vi "Json Token to Cluster Data.vi"(0 "Token Array":T1[](array[typedef]), 1 "Variable Names":string[](array[string]), 5 "Index":i32, 7 "Parent Ref In":refnum<vi>[](array[refnum]), 9 "Inception Tracking In":cluster{"In Array?":bool, "Cluster Level":i32}={"In Array?"=TRUE, "Cluster Level"=0}, 11 "Error In":errorcluster) -> (4 "index out":i32, 6 "Parent Ref Out":refnum<vi>[](array[refnum]), 10 "Inception Tracking Out":cluster{"In Array?":bool, "Cluster Level":i32}={"In Array?"=TRUE, "Cluster Level"=0}, 14 "End?":bool, 15 "Error Out":errorcluster)   [LabVIEW 2019, in "SLL JSON to Cluster.lvlib"]
doc: "This VI converts input JSON tokens to its equivalent cluster data"
uses:
  SLL JSON to Cluster.lvlib
  _Controls/Tokens.ctl
  <vilib>/numeric/LVNumericRepresentation.ctl
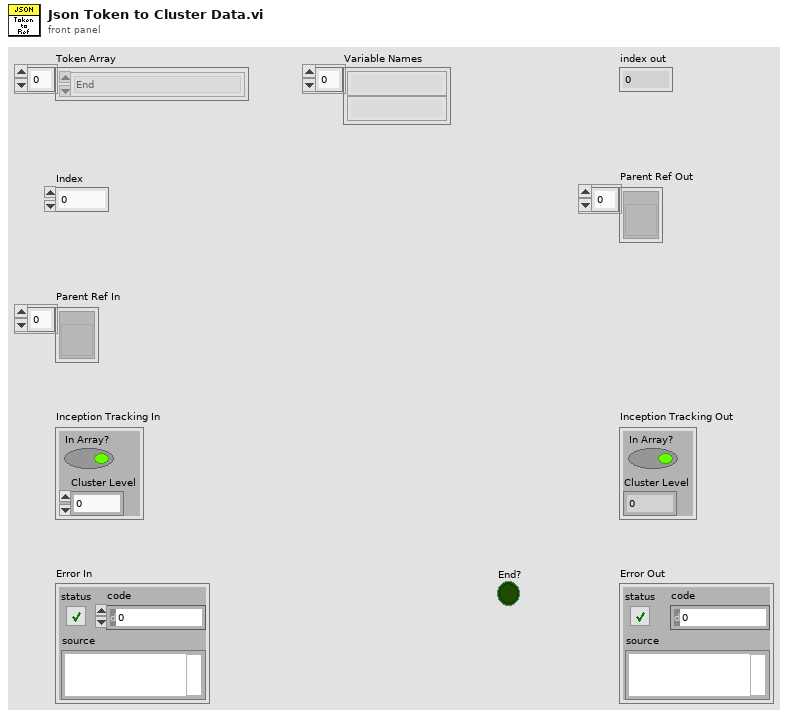
[diagram p1: front panel]
types:
  T1 = typedef "SLL JSON to Cluster.lvlib/Tokens.ctl" = enum16{"End", "Boolean", "Named Cluster", "Unnamed Cluster", "Array", "String", "Decimal", "FloatingPoint", "End Array", "End Cluster"}
  T2 = typedef "LVNumericRepresentation.ctl" = enum32{"Extended Precision", "Double Precision", "Single Precision", "Long", "Word", "Byte", "Unsigned Long", "Unsigned Word", "Unsigned Byte", "Complex Extended", "Complex Double", "Complex Single", "Quad", "Unsigned Quad", "Fixed-Point"}
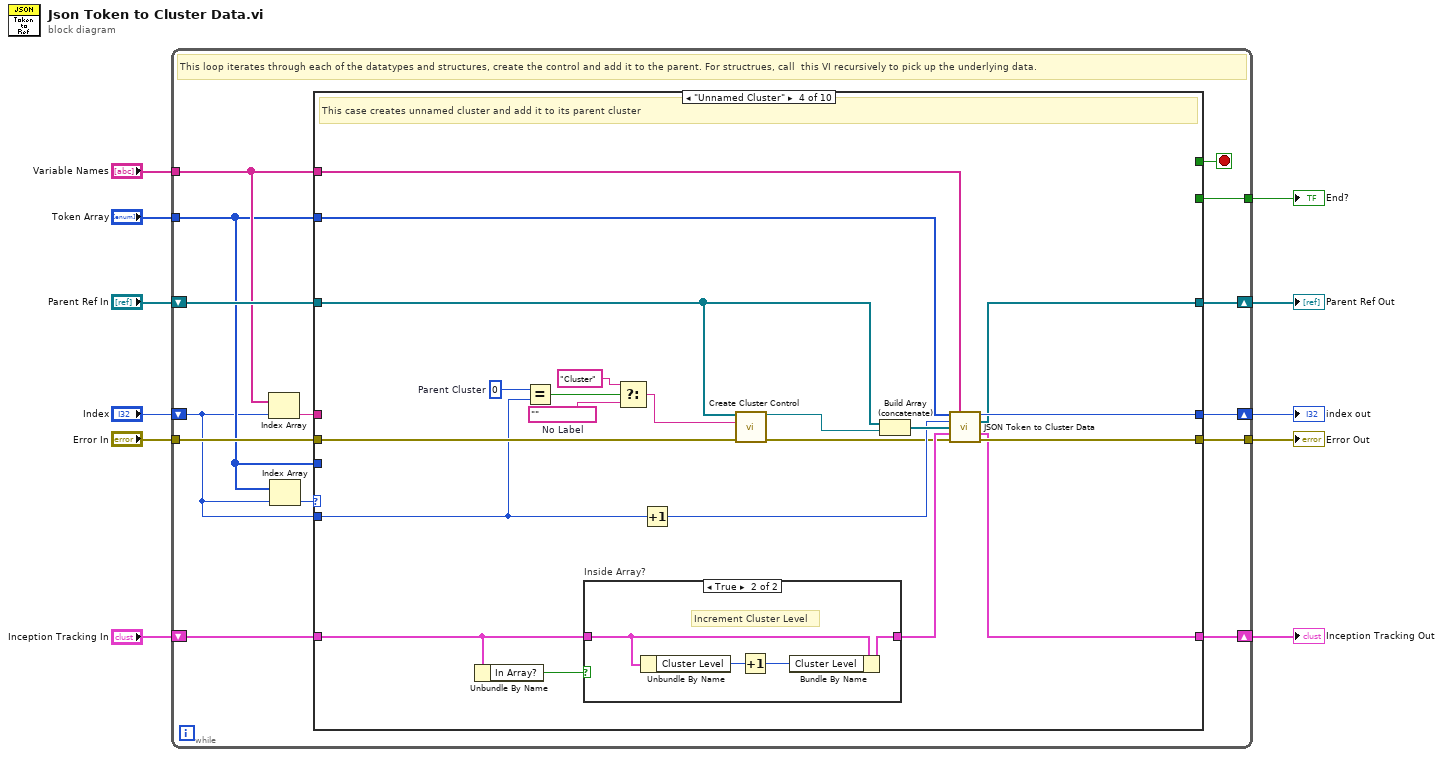
[diagram p0: block diagram]
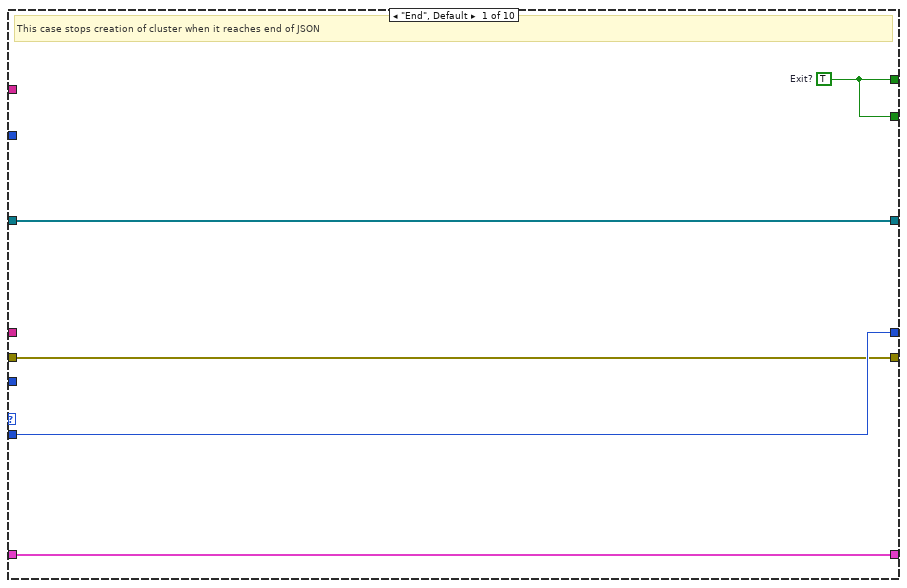
[diagram p2: hidden frame]
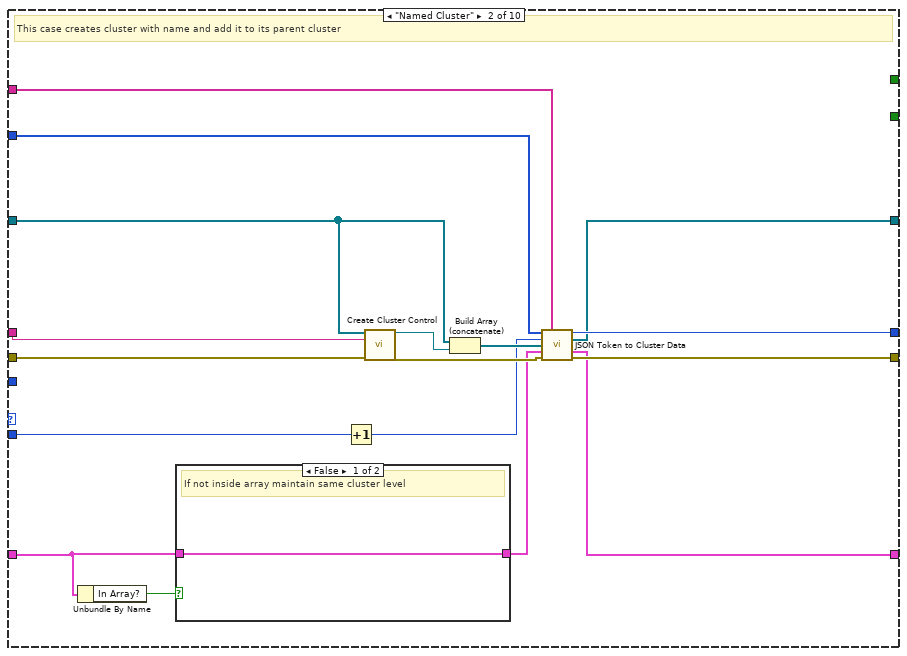
[diagram p3: hidden frame]
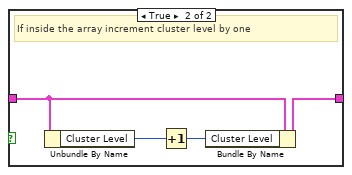
[diagram p4: hidden frame]
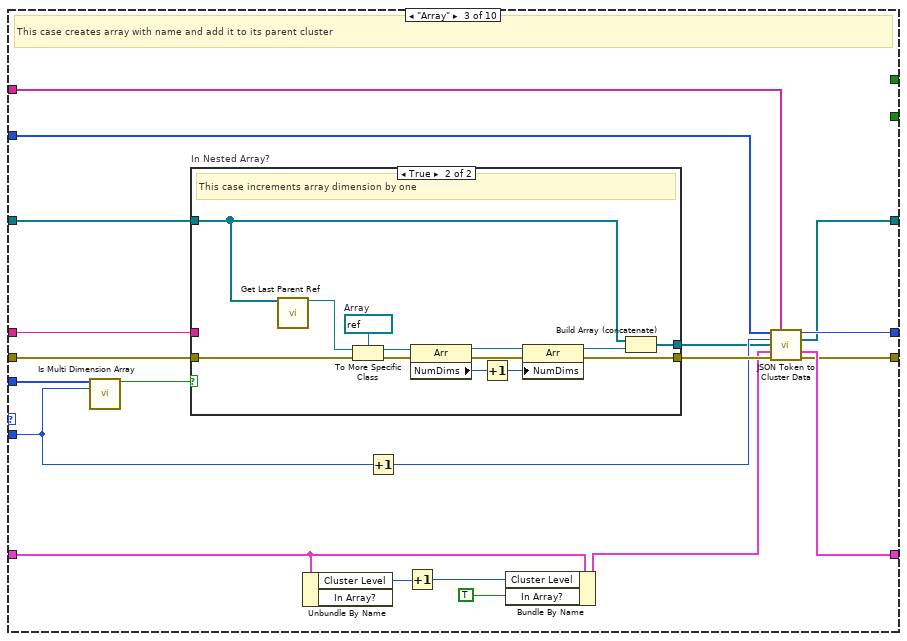
[diagram p5: hidden frame]
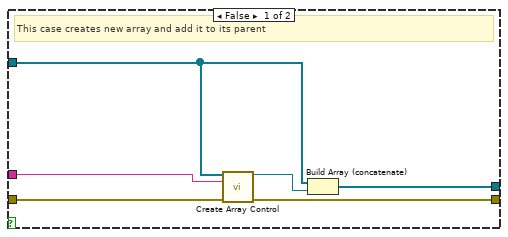
[diagram p6: hidden frame]
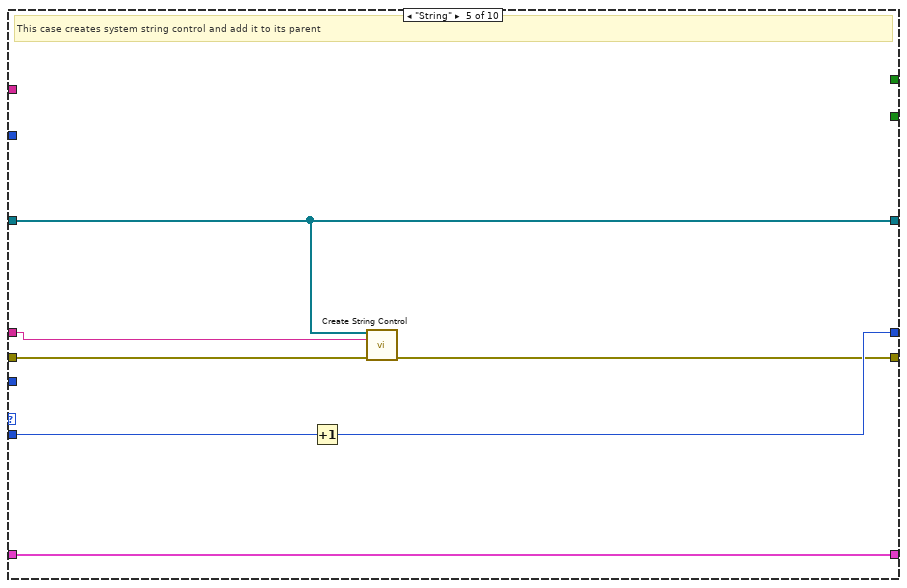
[diagram p8: hidden frame]
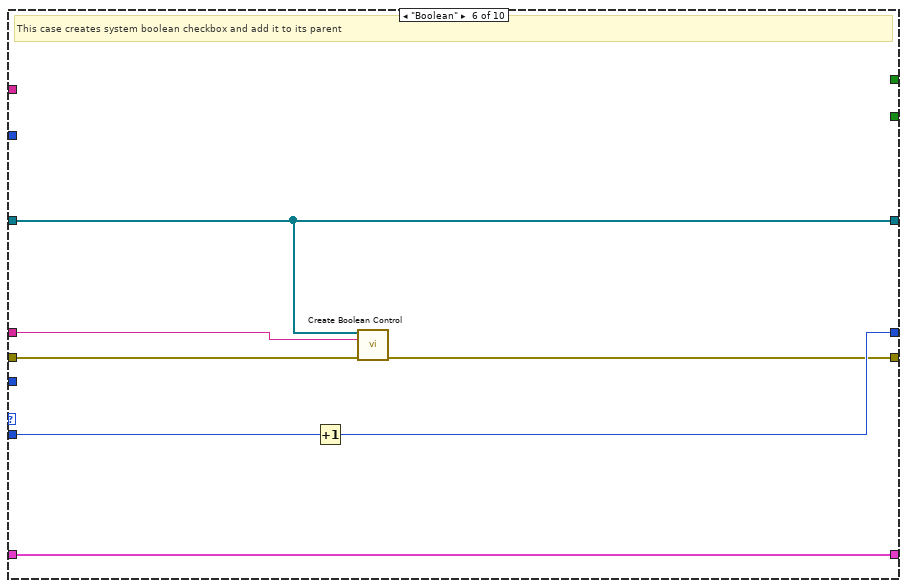
[diagram p9: hidden frame]
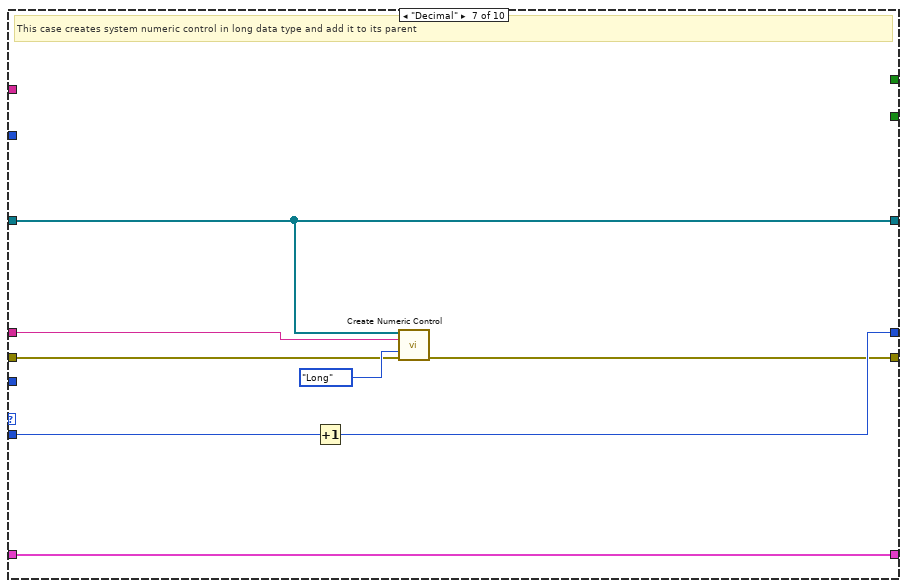
[diagram p10: hidden frame]
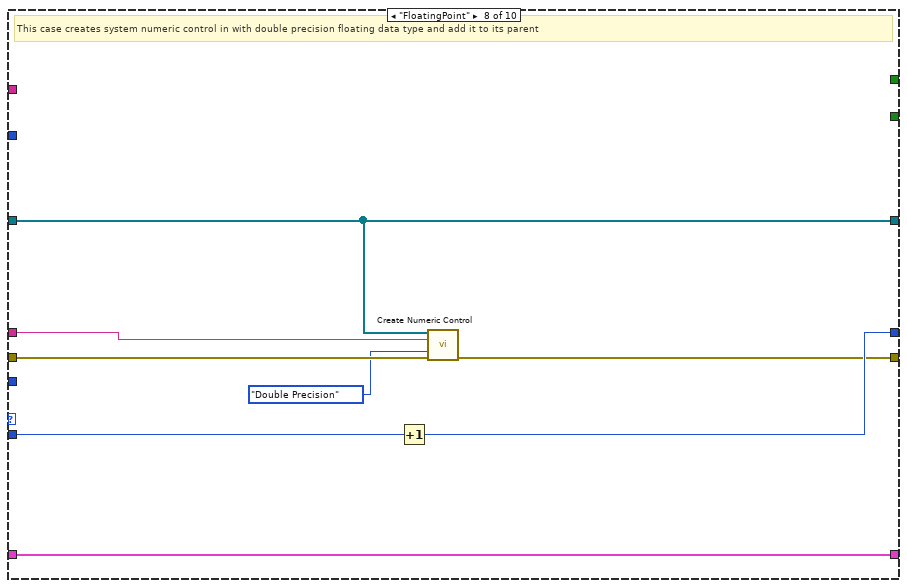
[diagram p11: hidden frame]
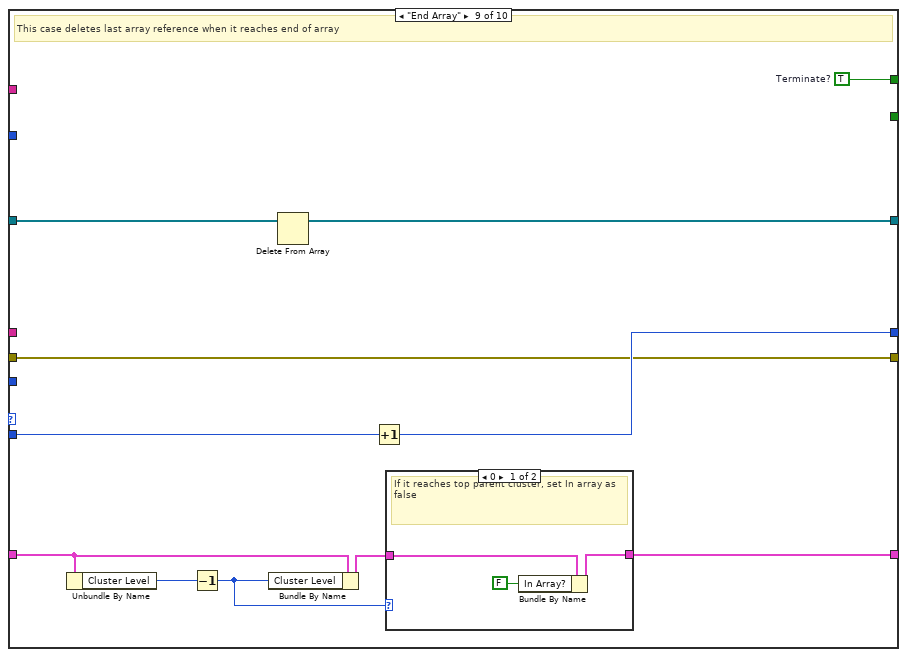
[diagram p12: hidden frame]
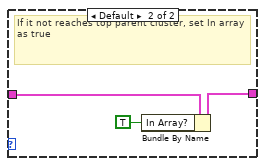
[diagram p13: hidden frame]
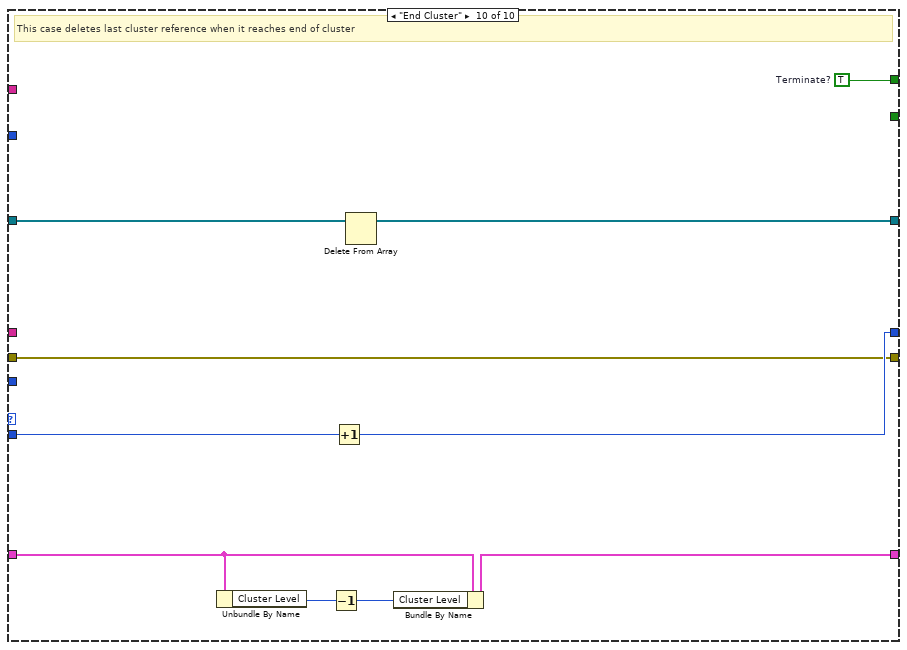
[diagram p14: hidden frame]
diagram:
  n1 = while {
    tunnel: "Token Array" -> [w13]
    shift-right: [w21] -> w9
    shift-left: "Index" -> [w12]
    shift-right: [w22] -> w4
    shift-left: "Parent Ref In" -> [w24]
    tunnel: "Variable Names" -> [w18]
    tunnel: [w19] -> w7
    shift-right: [w16] -> w5
    shift-left: "Inception Tracking In" -> [w17]
    tunnel: "Error In" -> [w15]
    tunnel: [w14] -> w1
    stop <- w20 stop-if-true
    # "This loop iterates through each of the datatypes and structures, create the control and add it to the parent. For structrues, call  this VI recursively to pick up the underlying data."
    n2 = Index Array(array=w18, index=w12) -> (element=w23:string)
    n3 = Index Array(array=w13, index=w12) -> (element=w25:T1)
    n4 = case shown="\"Unnamed Cluster\"" w25 {
      tunnel: w24 -> [w29 w43 w71 w100 w118 w125 w132 w141 w150 w167]
      tunnel: w23 -> [_ w46 w72 _ w124 w131 w137 w140 _ _]
      tunnel: [w29 w33 w61 w102 w118 w125 w132 w141 w149 w166] -> w22
      tunnel: w12 -> [w28 w47 w54 w97 w123 w130 w139 w147 w157 w173]
      tunnel: [w28 w34 w64 w104 w122 w129 w138 w146 w156 w172] -> w21
      tunnel: [w30 _ _ _ _ _ _ _ w158 w174] -> w20
      tunnel: [w30 _ _ _ _ _ _ _ _ _] -> w19
      tunnel: w13 -> [_ w35 w66 w108 _ _ _ _ _ _]
      tunnel: w18 -> [_ w31 w60 w105 _ _ _ _ _ _]
      tunnel: w17 -> [w27 w45 w59 w112 w121 w128 w135 w145 w154 w170]
      tunnel: [w27 w32 w63 w109 w121 w128 w135 w145 w151 w169] -> w16
      tunnel: w15 -> [w26 w41 w70 w101 w120 w127 w134 w144 w148 w165]
      tunnel: [w26 w39 w62 w110 w119 w126 w133 w143 w148 w165] -> w14
      tunnel: w13 -> [_ _ w58 _ _ _ _ _ _ _]
      frame "End", Default {
        w30 = TRUE  # Exit?
        # "This case stops creation of cluster when it reaches end of JSON"
      }
      frame "Named Cluster" {
        # "This case creates cluster with name and add it to its parent cluster"
        n5 = Unbundle By Name(w45) -> ("In Array?"=w44:bool)
        n6 = case shown="False" w44 {
          tunnel: [w48 w50] -> w38
          tunnel: w45 -> [w48 w49]
          frame False {
            # "If not inside array maintain same cluster level"
          }
          frame True {
            # "If inside the array increment cluster level by one"
            n7 = Unbundle By Name(w49) -> ("Cluster Level"=w52:i32)
            n8 = Increment(x=w52) -> (x+1=w51:i32)
            n9 = Bundle By Name(cluster=w49, "Cluster Level"=w51) -> (w50:cluster{"In Array?":bool, "Cluster Level":i32})
          }
        }
        n10 = Increment(x=w47) -> (x+1=w36:i32)
        n11 = call "Create Cluster Control.vi"("Parent Ref In"=w43, "Cluster Label"=w46, "Error In"=w41) -> ("Cluster Ref Out"=w42:refnum<vi>, "Error Out"=w40:errorcluster)  [unwired: 11 in]
        n12 = Build Array (concatenate)(w43, w42) -> (w37:refnum<vi>[])
        n13 = call "JSON Token to Cluster Data.vi"("Token Array"=w35, "Variable Names"=w31, "Index"=w36, "Parent Ref In"=w37, "Inception Tracking In"=w38, "Error In"=w40) -> ("index out"=w34:i32, "Parent Ref Out"=w33:refnum<vi>[], "Inception Tracking Out"=w32:cluster{"In Array?":bool, "Cluster Level":i32}, "Error Out"=w39:errorcluster)  [unwired: 5 in, 1 out]
      }
      frame "Array" {
        # "This case creates array with name and add it to its parent cluster"
        n14 = call "Is Multi Dimension Array.vi"("Token Array"=w58, "Previous Index"=w54) -> ("Is Nested Array?"=w53:bool)  [unwired: 13 in]
        n15 = case "In Nested Array?" shown="True" w53 {
          tunnel: w72 -> [w78 _]
          tunnel: w71 -> [w73 w80]
          tunnel: w70 -> [w76 w90]
          tunnel: [w75 w86] -> w69
          tunnel: [w74 w82] -> w65
          frame False {
            # "This case creates new array and add it to its parent"
            n16 = call "Create Array Control.vi"("Parent Ref In"=w73, "Array Label"=w78, "Error In"=w76) -> ("Array Ref Out"=w77:refnum<vi>, "Error Out"=w75:errorcluster)  [unwired: 11 in]
            n17 = Build Array (concatenate)(w73, w77) -> (w74:refnum<vi>[])
          }
          frame True {
            w88 = refnum<vi> refnum  # Array
            # "This case increments array dimension by one"
            n18 = call "Get Last Parent Ref.vi"("Parent Ref In"=w80) -> ("Last Parent Ref"=w79:refnum<vi>)  [unwired: 14 in]
            n19 = To More Specific Class(target class=w88, reference=w79, error in=w90) -> (specific class reference=w87:refnum<vi>, error out=w89:errorcluster)
            n20 = property class="Arr"(reference=w87, error in=w89) -> (reference out=w85:refnum<vi>, error out=w91:errorcluster, "NumDims"=w84:u32)
            n21 = Increment(x=w84) -> (x+1=w83:u32)
            n22 = property class="Arr"(reference=w85, error in=w91, "NumDims"=w83) -> (reference out=w81:refnum<vi>, error out=w86:errorcluster)
            n23 = Build Array (concatenate)(w80, w81) -> (w82:refnum<vi>[])
          }
        }
        n24 = Unbundle By Name(w59) -> ("Cluster Level"=w56:i32)  [unwired: 1 out]
        n25 = Increment(x=w54) -> (x+1=w68:i32)
        n26 = Increment(x=w56) -> (x+1=w55:i32)
        n27 = Bundle By Name(cluster=w59, "Cluster Level"=w55, "In Array?"=TRUE) -> (w67:cluster{"In Array?":bool, "Cluster Level":i32})
        n28 = call "JSON Token to Cluster Data.vi"("Token Array"=w66, "Variable Names"=w60, "Index"=w68, "Parent Ref In"=w65, "Inception Tracking In"=w67, "Error In"=w69) -> ("index out"=w64:i32, "Parent Ref Out"=w61:refnum<vi>[], "Inception Tracking Out"=w63:cluster{"In Array?":bool, "Cluster Level":i32}, "Error Out"=w62:errorcluster)  [unwired: 5 in, 1 out]
      }
      frame "Unnamed Cluster" {
        w96 = 0  # Parent Cluster
        w93 = ""  # No Label
        # "This case creates unnamed cluster and add it to its parent cluster"
        n29 = Unbundle By Name(w112) -> ("In Array?"=w111:bool)
        n30 = Equal?(x=w96, y=w97) -> (x = y?=w95:bool)
        n31 = case "Inside Array?" shown="True" w111 {
          tunnel: [w113 w115] -> w107
          tunnel: w112 -> [w113 w114]
          frame False {
          }
          frame True {
            # "Increment Cluster Level"
            n32 = Unbundle By Name(w114) -> ("Cluster Level"=w117:i32)
            n33 = Increment(x=w117) -> (x+1=w116:i32)
            n34 = Bundle By Name(cluster=w114, "Cluster Level"=w116) -> (w115:cluster{"In Array?":bool, "Cluster Level":i32})
          }
        }
        n35 = Select(t="Cluster", s=w95, f=w93) -> (s? t:f=w94:string)
        n36 = Increment(x=w97) -> (x+1=w103:i32)
        n37 = call "Create Cluster Control.vi"("Parent Ref In"=w100, "Cluster Label"=w94, "Error In"=w101) -> ("Cluster Ref Out"=w99:refnum<vi>, "Error Out"=w98:errorcluster)  [unwired: 11 in]
        n38 = Build Array (concatenate)(w100, w99) -> (w106:refnum<vi>[])
        n39 = call "JSON Token to Cluster Data.vi"("Token Array"=w108, "Variable Names"=w105, "Index"=w103, "Parent Ref In"=w106, "Inception Tracking In"=w107, "Error In"=w98) -> ("index out"=w104:i32, "Parent Ref Out"=w102:refnum<vi>[], "Inception Tracking Out"=w109:cluster{"In Array?":bool, "Cluster Level":i32}, "Error Out"=w110:errorcluster)  [unwired: 5 in, 1 out]
      }
      frame "String" {
        # "This case creates system string control and add it to its parent"
        n40 = Increment(x=w123) -> (x+1=w122:i32)
        n41 = call "Create String Control.vi"("Parent Ref In"=w118, "String Control label"=w124, "Error In"=w120) -> ("Error Out"=w119:errorcluster)  [unwired: 12 in]
      }
      frame "Boolean" {
        # "This case creates system boolean checkbox and add it to its parent"
        n42 = Increment(x=w130) -> (x+1=w129:i32)
        n43 = call "Create Boolean Control.vi"("Parent Ref In"=w125, "Boolean Label"=w131, "Error In"=w127) -> ("Error Out"=w126:errorcluster)  [unwired: 12 in]
      }
      frame "Decimal" {
        # "This case creates system numeric control in long data type and add it to its parent"
        n44 = Increment(x=w139) -> (x+1=w138:i32)
        n45 = call "Create Numeric Control.vi"("Parent Ref In"=w132, "Control Label"=w137, "Representation"=LVNumericRepresentation."Long", "Error In"=w134) -> ("Error Out"=w133:errorcluster)  [unwired: 11 in]
      }
      frame "FloatingPoint" {
        # "This case creates system numeric control in with double precision floating data type and add it to its parent"
        n46 = Increment(x=w147) -> (x+1=w146:i32)
        n47 = call "Create Numeric Control.vi"("Parent Ref In"=w141, "Control Label"=w140, "Representation"=LVNumericRepresentation."Double Precision", "Error In"=w144) -> ("Error Out"=w143:errorcluster)  [unwired: 11 in]
      }
      frame "End Array" {
        w158 = TRUE  # Terminate?
        # "This case deletes last array reference when it reaches end of array"
        n48 = Unbundle By Name(w154) -> ("Cluster Level"=w155:i32)
        n49 = Decrement(x=w155) -> (x-1=w152:i32)
        n50 = Bundle By Name(cluster=w154, "Cluster Level"=w152) -> (w153:cluster{"In Array?":bool, "Cluster Level":i32})
        n51 = Delete From Array(array=w150) -> (array with subset deleted=w149:refnum<vi>[])  [unwired: 2 in, 1 out]
        n52 = Increment(x=w157) -> (x+1=w156:i32)
        n53 = case "Inside parent cluster" shown="0" w152 {
          tunnel: w153 -> [w161 w164]
          tunnel: [w159 w162] -> w151
          frame 0 {
            # "If it reaches top parent cluster, set In array as false"
            n54 = Bundle By Name(cluster=w161, "In Array?"=FALSE) -> (w159:cluster{"In Array?":bool, "Cluster Level":i32})
          }
          frame Default {
            # "If it not reaches top parent cluster, set In array as true"
            n55 = Bundle By Name(cluster=w164, "In Array?"=TRUE) -> (w162:cluster{"In Array?":bool, "Cluster Level":i32})
          }
        }
      }
      frame "End Cluster" {
        w174 = TRUE  # Terminate?
        # "This case deletes last cluster reference when it reaches end of cluster"
        n56 = Unbundle By Name(w170) -> ("Cluster Level"=w171:i32)
        n57 = Decrement(x=w171) -> (x-1=w168:i32)
        n58 = Increment(x=w173) -> (x+1=w172:i32)
        n59 = Delete From Array(array=w167) -> (array with subset deleted=w166:refnum<vi>[])  [unwired: 2 in, 1 out]
        n60 = Bundle By Name(cluster=w170, "Cluster Level"=w168) -> (w169:cluster{"In Array?":bool, "Cluster Level":i32})
      }
    }
  }
  "index out" <- w9
  "End?" <- w7
  "Inception Tracking Out" <- w5
  "Parent Ref Out" <- w4
  "Error Out" <- w1
